vi "Flatten UIP Value.vi"(11 "FontUIP In":refnum<class "FontUIP.lvclass">) -> (0 "Error Out":errorcluster, 2 "String Value":string, 3 "FontUIP Out":refnum<class "FontUIP.lvclass">)   [LabVIEW 2016, in "FontUIP.lvclass"]
doc: "Overwrite this abstract method to implement child behavior for flattening the UIP private data into XML compatible string format."
uses:
  FontUIP.lvclass
  FontUIP.lvclass/FontUIP.ctl
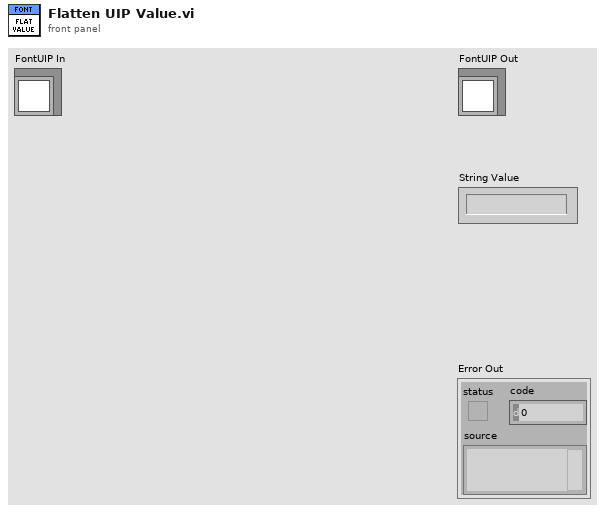
[diagram p1: front panel]
types:
  T1 = typedef "LVFontTypeDef.ctl" = cluster{"Font Name":string, "Size":u16, "Bold":bool, "Italic":bool, "Underline":bool, "Strikeout":bool, "Color":u32}
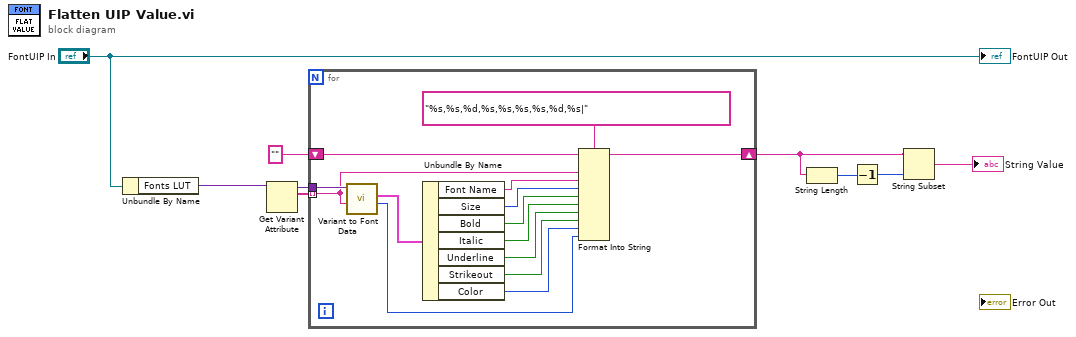
[diagram p0: block diagram]
diagram:
  n1 = Unbundle By Name("FontUIP In") -> ("Fonts LUT"=w8:variant)
  n2 = Get Variant Attribute(Variant=w8) -> (duplicate Variant=w5:variant, names=w6:string[])  [unwired: 3 in, 2 out]
  n3 = for {
    shift-right: [w21] -> w3
    shift-left: "" -> [w22]
    tunnel: w6 -> [w10] mode=indexing
    tunnel: w5 -> [w23]
    n4 = call "Variant to Font Data.vi"("Font Key Name"=w10, "Fonts LUT in"=w23) -> ("Justification"=w11:enum16{"Left", "Center", "Right"}, "Font"=w20:T1)  [unwired: 6 in, 2 out]
    n5 = Unbundle By Name(w20) -> ("Font Name"=w19:string, "Size"=w18:u16, "Bold"=w17:bool, "Italic"=w16:bool, "Underline"=w15:bool, "Strikeout"=w14:bool, "Color"=w13:u32)
    n6 = Format Into String(format string="%s,%s,%d,%s,%s,%s,%s,%d,%s|", initial string=w22, w10, w19, w18, w17, w16, w15, w14, w13, w11) -> (resulting string=w21:string)  [unwired: 1 in, 1 out]
  }
  n7 = String Length(string=w3) -> (length=w4:i32)
  n8 = Decrement(x=w4) -> (x-1=w2:i32)
  n9 = String Subset(string=w3, length (rest)=w2) -> (substring=→"String Value":string)  [unwired: 1 in]
  "FontUIP Out" <- "FontUIP In"
